vi "Hab Driver TeleOp.vi"(11 "Controller Values":T1) -> ()   [LabVIEW 2018]
uses:
  Support Code/Controller Values.ctl
  <vilib>/Rock Robotics/Network Tables/NT Read Boolean.vi
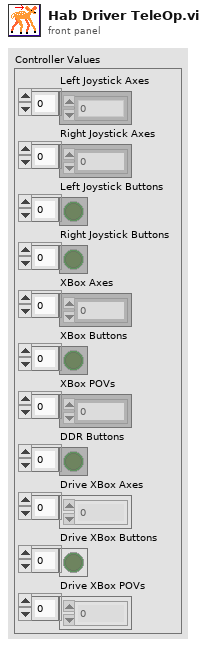
[diagram p1: front panel]
types:
  T1 = typedef "Controller Values.ctl" = cluster{"Left Joystick Axes ":dbl[], "Right Joystick Axes":dbl[], "Left Joystick Buttons":bool[], "Right Joystick Buttons":bool[], "XBox Axes":dbl[], "XBox Buttons":bool[], "XBox POVs":i16[], "DDR Buttons":bool[], "Drive XBox Axes":dbl[], "Drive XBox Buttons":bool[], "Drive XBox POVs":i16[]}
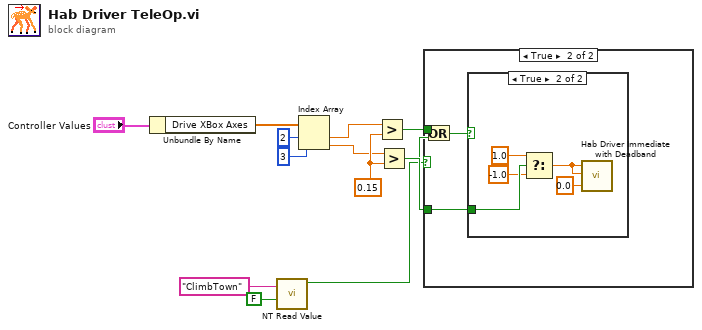
[diagram p0: block diagram]
diagram:
  w11 = 0.15 ("y")
  n1 = Unbundle By Name("Controller Values") -> ("Drive XBox Axes"=w10:dbl[])
  n2 = call-poly <vilib>:"NT Read Value.vi"("Default Value"=FALSE, "Name"="ClimbTown") -> ("Boolean"=w3:bool)  [unwired: 8 in, 1 out]
  n3 = Index Array(array=w10, index #1=2 ("index"), index #2=3 ("index")) -> (element #1=w4:dbl, element #2=w7:dbl)
  n4 = Greater?(x=w4, y=w11) -> (0:w5:bool)
  n5 = Greater?(x=w7, y=w11) -> (0:w6:bool)
  n6 = case shown="True" w3 {
    tunnel: w6 -> [_ w14]
    tunnel: w5 -> [_ w13]
    frame False {
    }
    frame True {
      n7 = Or(x=w13, y=w14) -> (x .or. y?=w15:bool)
      n8 = case shown="True" w15 {
        tunnel: w14 -> [_ w20]
        frame False {
        }
        frame True {
          n9 = Select(t=1.0, s=w20, f=-1.0) -> (s? t:f=w17:dbl)
          n10 = call "Hab Driver Immediate with Deadband.vi"("Deadband Value"=0.0, "Right Setpoint"=w17, "Left Setpoint"=w17) -> ()  [unwired: 8 in, 1 out]
        }
      }
    }
  }
